vi "Auto Save DAQ.vi"() -> ()   [LabVIEW 2010]
uses:
  <vilib>/Utility/file.llb/Write To Spreadsheet File (I64).vi
panel:
  out "Peak to Peak Diff":u16
  in  "Auto Save Data":bool=TRUE
  out "date/time string":string="2012-02-20 12-35.08"
  in  "time format string (%c)":string="%Y-%m-%d %H-%M.%S"
  in  "Data file path ending":string=".dat"
  out "Previous acquisition":u16[](graph)
  in  "LowChan":i32
  in  "HighChan":i32
  in  "Count":i32=1000
  in  "Rate":i32=3000
  out "Current acquisition":u16[](graph)
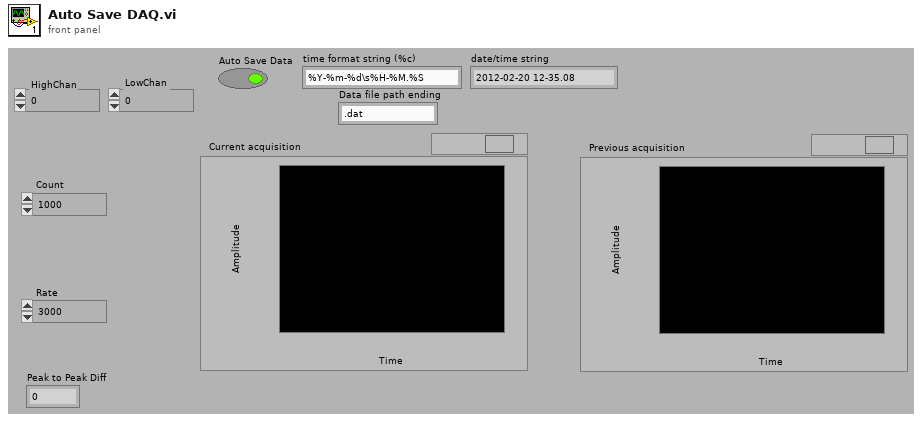
[diagram p1: front panel]
types:
  T1 = typedef "imagedata.ctl" = cluster{"image type":i32, "image depth":i32, "image":u8[], "mask":u8[], "colors":u32[], "Rectangle":cluster{"left":i16, "top":i16, "right":i16, "bottom":i16}}
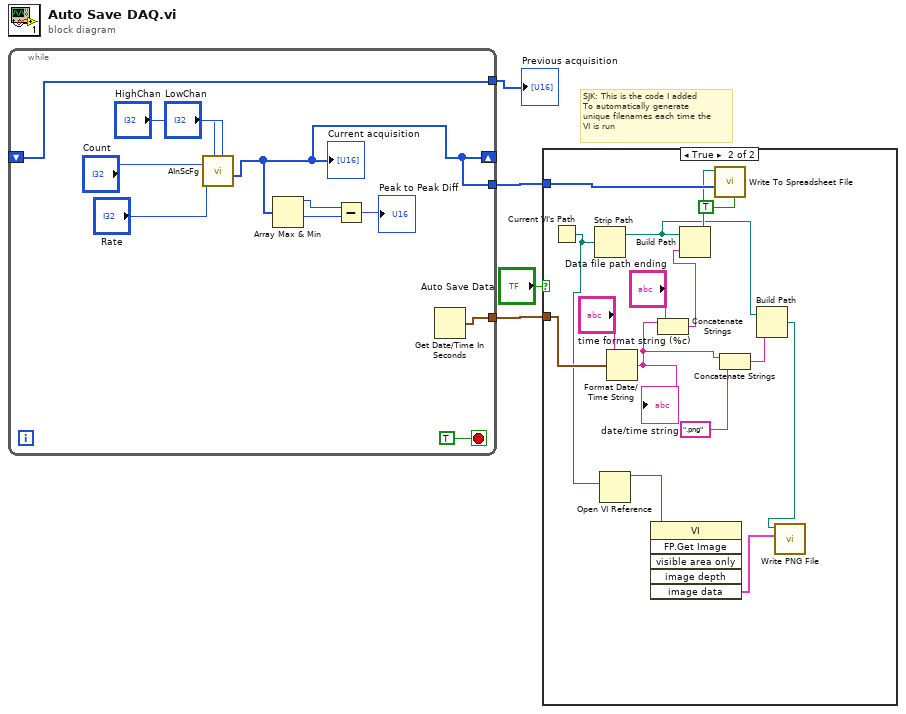
[diagram p0: block diagram]
diagram:
  # "SJK: This is the code I added\nTo automatically generate \nunique filenames each time the\nVI is run"
  n1 = while {
    shift-right: [w8] -> _
    shift-left: _ -> [w10]
    tunnel: [w10] -> w4
    tunnel: [w8] -> w3
    tunnel: [w9] -> w2
    stop <- TRUE stop-if-true
    n2 = call <menus>:"AInScFg.VI"("LowChan"="LowChan", "HighChan"="HighChan", "Rate"="Rate", "Count"="Count") -> ("ADData"=w8:u16[])  [unwired: 4 in, 2 out]
    "Current acquisition" <- w8
    n3 = Array Max & Min(array=w8) -> (max value=w7:u16, min value=w6:u16)  [unwired: 2 out]
    n4 = Subtract(x=w7, y=w6) -> (x-y=→"Peak to Peak Diff":u16)
    n5 = Get Date/Time In Seconds() -> (seconds since 1Jan1904=w9:timestamp)
  }
  "Previous acquisition" <- w4
  n6 = case shown="True" "Auto Save Data" {
    tunnel: w3 -> [_ w30]
    tunnel: w2 -> [_ w29]
    frame False {
    }
    frame True {
      n7 = Current VI's Path() -> (path=w21:path)
      n8 = Strip Path(path=w21) -> (stripped path=w20:path)  [unwired: 1 out]
      n9 = Open VI Reference(vi path=w21) -> (vi reference=w22:refnum<vi>)  [unwired: 5 in, 1 out]
      n10 = Format Date/Time String(time format string (%c)="time format string (%c)", seconds (now)=w29) -> (date/time string=w19:string)  [unwired: 1 in]
      "date/time string" <- w19
      n11 = invoke class="VI" method="FP.Get Image"(reference=w22) -> ("image data"=w23:T1)  [unwired: 5 in, 5 out]
      n12 = Concatenate Strings(w19, "Data file path ending") -> (w26:string)
      n13 = Build Path(base path=w20, name or relative path=w26) -> (appended path=w25:path)
      n14 = call-poly <vilib>:"Write To Spreadsheet File.vi"("transpose? (no:F)"=TRUE, "1D data"=w30, "file path (dialog if empty)"=w25) -> ()  [unwired: 5 in, 1 out]
      n15 = Concatenate Strings(w19, ".png" ("string")) -> (w17:string)
      n16 = Build Path(base path=w20, name or relative path=w17) -> (appended path=w16:path)
      n17 = call <vilib>:"Write PNG File.vi"("image data"=w23, "path to PNG file"=w16) -> ()  [unwired: 8 in, 2 out]
    }
  }
